vi "deviceSearchResponse.vi"(5 "port or service name":u16, 7 "address":u32, 8 "error in (no error)":errorcluster, 9 "root":T1, 10 "datain":string, 11 "connection ID":refnum<k16>) -> (0 "error out":errorcluster, 3 "connection ID out":refnum<k16>)   [LabVIEW 2010]
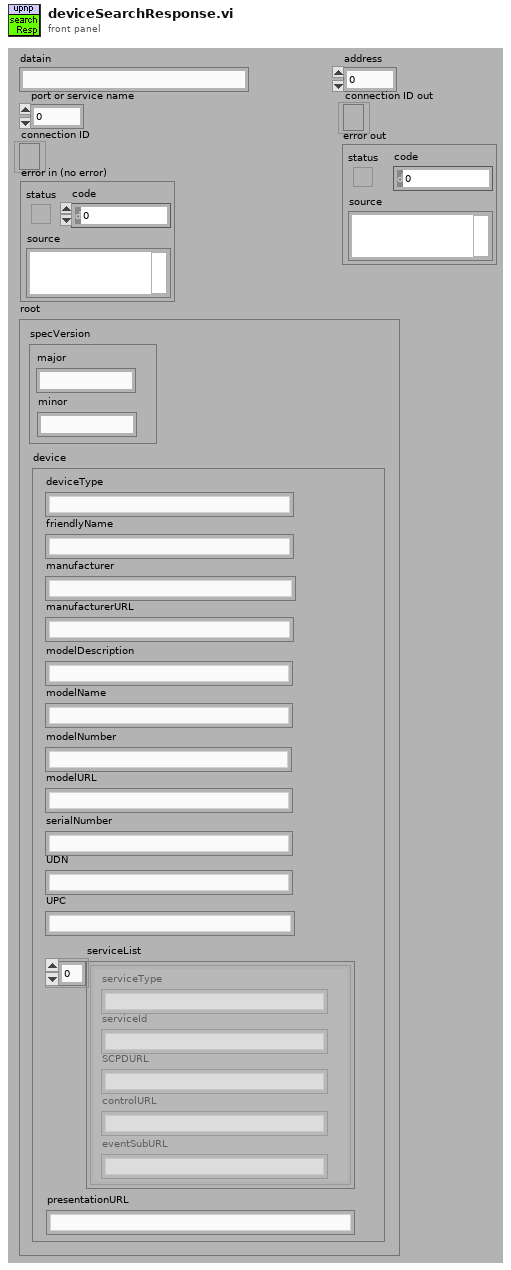
[diagram p1: front panel]
types:
  T1 = cluster{"specVersion":cluster{"major":string, "minor":string}, "device":cluster{"deviceType":string, "friendlyName":string, "manufacturer":string, "manufacturerURL":string, "modelDescription":string, "modelName":string, "modelNumber":string, "modelURL":string, "serialNumber":string, "UDN":string, "UPC":string, "serviceList":cluster{"serviceType":string, "serviceId":string, "SCPDURL":string, "controlURL":string, "eventSubURL":string}[], "presentationURL":string}}
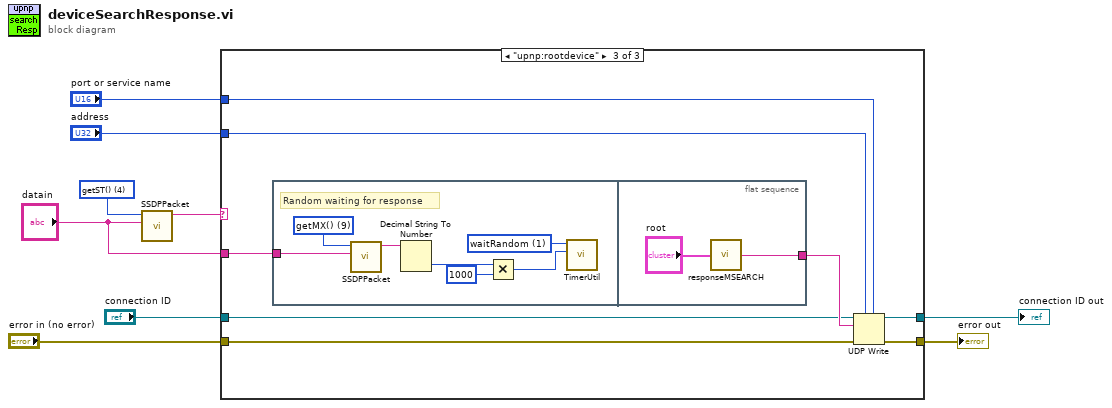
[diagram p0: block diagram]
diagram:
  w9 = u16 4 items=["getHost()", "getCacheControl()", "getLocation()", "getMAN()", "getST()", "getNT()", "getNTS()", "getServer()", "getUSN()", "getMX()"] ("getMethods")
  n1 = call "SSDPPacket.vi"("data"="datain", "getMethods"=w9) -> ("value"=w8:string)  [unwired: 9 out]
  n2 = case shown="\"upnp:rootdevice\"" w8 {
    tunnel: "port or service name" -> [_ _ w20]
    tunnel: "address" -> [_ _ w19]
    tunnel: "datain" -> [_ _ w18]
    tunnel: "connection ID" -> [w11 w13 w17]
    tunnel: [w11 w13 w16] -> w3
    tunnel: "error in (no error)" -> [w10 w12 w15]
    tunnel: [w10 w12 w14] -> w1
    frame "", Default {
    }
    frame "ssdp:all" {
    }
    frame "upnp:rootdevice" {
      n3 = flat-sequence {
        tunnel: w18 -> [w22]
        tunnel: [w30] -> w21
        frame #0 {
          w26 = u16 1 items=["wait", "waitRandom"] ("typeTimer")
          w28 = u16 9 items=["getHost()", "getCacheControl()", "getLocation()", "getMAN()", "getST()", "getNT()", "getNTS()", "getServer()", "getUSN()", "getMX()"] ("getMethods")
          # "Random waiting for response"
          n4 = call "SSDPPacket.vi"("data"=w22, "getMethods"=w28) -> ("value"=w27:string)  [unwired: 9 out]
          n5 = Decimal String To Number(string=w27) -> (number=w25:i32)  [unwired: 3 out]
          n6 = Multiply(x=w25, y=1000) -> (x*y=w23:i32)
          n7 = call "TimerUtil.vi"("time (msec)"=w23, "typeTimer"=w26) -> ()  [unwired: 10 out]
        }
        frame #1 {
          n8 = call "responseMSEARCH.vi"("root"="root") -> ("ucastResponseMSG"=w30:string)
        }
      }
      n9 = UDP Write(address=w19, port or service name=w20, connection ID=w17, data in=w21, 8:w15) -> (error out=w14:errorcluster, 3:w16:refnum<k16>)  [unwired: 1 out]
    }
  }
  "connection ID out" <- w3
  "error out" <- w1
